vi "ADC SNR_input_sweep.vi"(8 "error in (no error)":errorcluster, 9 "Sequence parameters":string[][](array[string])=[["Min limit", "Max limit", "Register sheet file", "Register Sheet"], ["", "", "CC2600.xls", "TX_BLE;Trim"], ["Reg write (addr;value)", "Operating frequency [Hz]", "", ""], ["NA", "2.44G", "", ""]], 10 "Run type":i32, 11 "Method parameters":T3={"Dev"={"Do not disturb DUT"=FALSE, "XOSC"=32000000.0, "Board type"="", "EM"="", "Configure tempboard"=TRUE, "Device specific info"=[], "Generic Object"=refnum}, "Method"={"Run type"=1, "Test name"="Current LPM2 4", "Comment"="", "Results folder"="", "AFC"=enum."Off", "Method name"="Current LPM2 4", "Method results"={"Excel brief report"=FALSE, "Spotfire report"=FALSE, "Starfish report"=FALSE}, "Operator"="", "Reference time"=timestamp(0 s since 1904-01-01), "AFC delay"=0.0, "Initialization"=enum."Enabled", "MD5 Sum"="", "HW addon board"=enum."None", "AFC Regsheet"="", "AFC Regfile"=path "", "dummy"=0.0}, "Inst"={"Instr"={"PS1"={"Name"="", "GPIB address"="", "VISA session"=""}, "PS2"={"Name"="", "GPIB address"="", "VISA session"=""}, "TC1"={"Name"="", "GPIB address"="", "VISA session"=""}, "TC2"={"Name"="", "GPIB address"="", "VISA session"=""}, "SA1"={"Name"="", "GPIB address"="", "VISA session"=""}, "SA2"={"Name"="", "GPIB address"="", "VISA session"=""}, "SG1"={"Name"="", "GPIB address"="", "VISA session"=""}, "SG2"={"Name"="", "GPIB address"="", "VISA session"=""}, "SG3"={"Name"="", "GPIB address"="", "VISA session"=""}, "MI1"={"Name"="", "GPIB address"="", "VISA session"=""}, "MI2"={"Name"="", "GPIB address"="", "VISA session"=""}, "SW SA"={"Name"="", "Controller addr"=""}, "SW SG"={"Name"="", "Controller addr"=""}, "MI3"={"Name"="", "GPIB address"="", "VISA session"=""}}, "Switchbox"={"RF Path"=0, "Cal compensation"=enum."TX", "Switchbox gain mode"="", "State"=enum."TX"}, "Instr to control (i.e. SA1)"="Default", "Intrument info string"=""}, "Sequence parameters"=[["Weight", "Min Limit", "Max Limit", "Register Sheet", "", "", "", "", "", "", "", "", ""], ["Vital", "", "1", "LPM2", "", "", "", "", "", "", "", "", ""], ["Resolution", "Reg write (addr;value)", "Chip mode", "Range", "", "", "", "", "", "", "", "", ""], ["u", "NA", "", "auto", "", "", "", "", "", "", "", "", ""]], "Cond"={"Temp logged"=25.0, "VDD1_PS1_6V"=-999.0, "VDD2_PS1_25V"=-999.0, "VDD4_PS2_25V"=-999.0, "VDD3_PS2_6V"=-999.0}, "Meas config"={"X-axis inner loop index"=32000000, "Y-axis outer loop index"=32000000, "X-axis"=[], "Y-axis"=[], "X-axis array req size"=32000000, "Y-axis array req size"=32000000, "Param description"=[], "Use meas clust for reporting"=FALSE, "Parameter index (page)"=0, "X-axis name"="", "Y-axis name"=""}} {"Cond"."VDD3_PS2_6V" format="%.3f"; "Cond"."VDD4_PS2_25V" format="%.3f"; "Cond"."VDD2_PS1_25V" format="%.3f"; "Cond"."VDD1_PS1_6V" format="%.3f"; "Method"."dummy" format="%.1p"; "Method"."AFC delay" format="%.1p"; "Dev"."XOSC" format="%.3p"}) -> (0 "error out":errorcluster, 1 "End method error":T2, 2 "Short Results":string[](array[string])=["0.00", "0.00", "0.00", "0.00"], 3 "Result summary":string[][](array[string])=[["Critical", "Output Power@2405 MHz", "-3", "4", "dBm"], ["Critical", "Output Power@2410 MHz", "-3", "4", "dBm"]])   [LabVIEW 2019]
doc: "[AutoDocStart]Performs crystal accuracy measurements. Measures the offset from ideal frequency. Primarily used for tuning XOSC capacitors and verifying XOSC trims.\n\nSweeping parameters: operating frequency, OSC override value and VDDR level\n\nResults: Offset frequency in ppm[AutoDocEnd]"
uses:
  User Lib/Utilities/Cluster definitions/Method input.ctl
  User Lib/Utilities/Cluster definitions/Device specific info.ctl
  User Lib/Utilities/Controls/Automatic Frequency Compensation types.ctl
  User Lib/Utilities/Controls/Method Reports.ctl
  User Lib/Utilities/Cluster definitions/Method Initialization.ctl
  User Lib/Utilities/Controls/HW addon boards.ctl
  User Lib/Utilities/Cluster definitions/Instr clust.ctl
  User Lib/Utilities/Switchbox control/SwitchBox_State._ENUMctl.ctl
  User Lib/Utilities/Cluster definitions/End method error cluster.ctl
  User Lib/Utilities/Cluster definitions/DUT vdd control.ctl
  User Lib/Utilities/Cluster definitions/DUT VDD4.ctl
  User Lib/Utilities/Cluster definitions/DUT VDD3.ctl
  User Lib/Utilities/Cluster definitions/DUT VDD2.ctl
  User Lib/Utilities/Cluster definitions/DUT VDD1.ctl
  35ec0895-51f9-4de3-b2a6-381c8b522c68.vi
  a1a5dd50-ef75-4989-863a-e44a6a63b90e.vi
  3a26386c-adf8-4bfd-9313-23d3b8777f38.vi
panel:
  in  "Tab Control":T1(tab)
  # "°C"
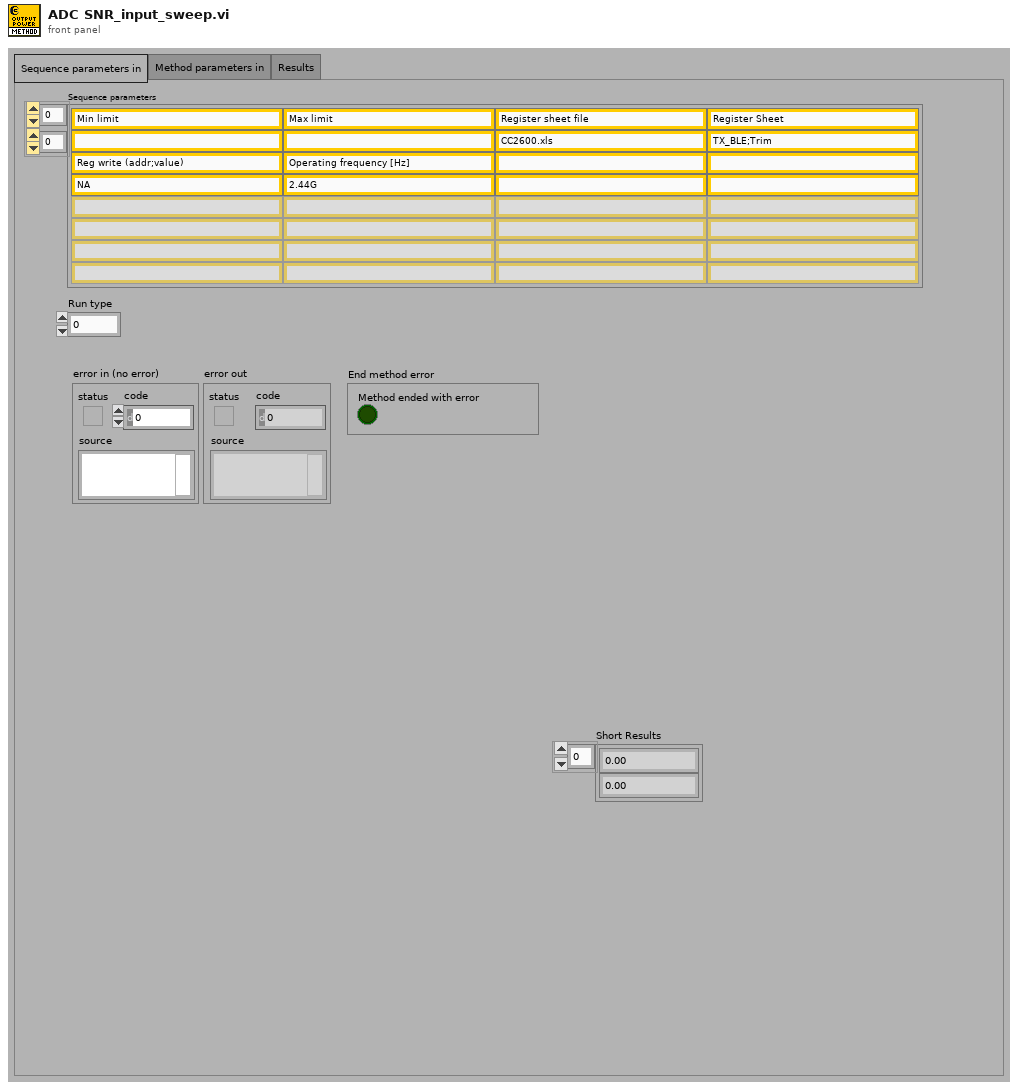
[diagram p1: front panel]
types:
  T1 = enum32{"Sequence parameters in", "Method parameters in", "Results"}
  T2 = typedef "End method error cluster.ctl" = cluster{"Method ended with error":bool}
  T3 = typedef "Method input.ctl" = cluster{"Dev":cluster{"Do not disturb DUT":bool, "XOSC":dbl, "Board type":string, "EM":string, "Configure tempboard":bool, "Device specific info":T4[], "Generic Object":refnum<class>}, "Method":cluster{"Run type":i32, "Test name":string, "Comment":string, "Results folder":string, "AFC":T5, "Method name":string, "Method results":T6, "Operator":string, "Reference time":timestamp, "AFC delay":dbl, "Initialization":T7, "MD5 Sum":string, "HW addon board":T8, "AFC Regsheet":string, "AFC Regfile":path, "dummy":dbl}, "Inst":T9, "Sequence parameters":string[][], "Cond":cluster{"Temp logged":dbl, "VDD1_PS1_6V":dbl, "VDD2_PS1_25V":dbl, "VDD4_PS2_25V":dbl, "VDD3_PS2_6V":dbl}, "Meas config":cluster{"X-axis inner loop index":i32, "Y-axis outer loop index":i32, "X-axis":string[], "Y-axis":string[], "X-axis array req size":i32, "Y-axis array req size":i32, "Param description":string[][], "Use meas clust for reporting":bool, "Parameter index (page)":i32, "X-axis name":string, "Y-axis name":string}}
  T4 = typedef "Device specific info.ctl" = cluster{"EM number":u8, "IP address":string, "Enabled":bool, "Slot no":u8, "RF path":u8, "EM name":string, "Wafer info":string, "AFC frequency ppm":dbl, "Register writes":string[][], "Meas data":string[][][], "Device comment":string}
  T5 = typedef "Automatic Frequency Compensation types.ctl" = enum16{"Off", "Compensate Instrument frequency", "Compensate DUT frequency", "Predictive - Compensate Instrument frequency", "Predictive - Compensate DUT frequency", "Do not skip re-init - Compensate Instrument frequency", "Do not skip re-init - Compensate DUT frequency"}
  T6 = typedef "Method Reports.ctl" = cluster{"Excel brief report":bool, "Spotfire report":bool, "Starfish report":bool}
  T7 = typedef "Method Initialization.ctl" = enum16{"Enabled", "Skip Instr and Device Init", "Enabled with Separate Flash", "Set PS, Device Init and Skip Instr Init", "Skip Device Init"}
  T8 = typedef "HW addon boards.ctl" = enum16{"None", "Current meas 5EM", "Stresstest 10EM"}
  T9 = typedef "Instr clust.ctl" = cluster{"Instr":cluster{"PS1":cluster{"Name":string, "GPIB address":string, "VISA session":refnum<visa-resource-name>}, "PS2":cluster{"Name":string, "GPIB address":string, "VISA session":refnum<visa-resource-name>}, "TC1":cluster{"Name":string, "GPIB address":string, "VISA session":refnum<visa-resource-name>}, "TC2":cluster{"Name":string, "GPIB address":string, "VISA session":refnum<visa-resource-name>}, "SA1":cluster{"Name":string, "GPIB address":string, "VISA session":refnum<visa-resource-name>}, "SA2":cluster{"Name":string, "GPIB address":string, "VISA session":refnum<visa-resource-name>}, "SG1":cluster{"Name":string, "GPIB address":string, "VISA session":refnum<visa-resource-name>}, "SG2":cluster{"Name":string, "GPIB address":string, "VISA session":refnum<visa-resource-name>}, "SG3":cluster{"Name":string, "GPIB address":string, "VISA session":refnum<visa-resource-name>}, "MI1":cluster{"Name":string, "GPIB address":string, "VISA session":refnum<visa-resource-name>}, "MI2":cluster{"Name":string, "GPIB address":string, "VISA session":refnum<visa-resource-name>}, "SW SA":cluster{"Name":string, "Controller addr":string}, "SW SG":cluster{"Name":string, "Controller addr":string}, "MI3":cluster{"Name":string, "GPIB address":string, "VISA session":refnum<visa-resource-name>}}, "Switchbox":cluster{"RF Path":i32, "Cal compensation":enum16{"TX", "RX", "Interferer", "No compensation", "Interferer2"}, "Switchbox gain mode":string, "State":T10}, "Instr to control (i.e. SA1)":string, "Intrument info string":string}
  T10 = typedef "SwitchBox_State._ENUMctl.ctl" = enum16{"TX", "RX", "SP:TX", "SP:RX", "SW:TX", "SW:RX"}
  T11 = typedef "DUT vdd control.ctl" = cluster{"VDD4 config":T12, "VDD3 config":T13, "VDD2 config":T14, "VDD1 config":T15}
  T12 = typedef "DUT VDD4.ctl" = u16
  T13 = typedef "DUT VDD3.ctl" = u16
  T14 = typedef "DUT VDD2.ctl" = u16
  T15 = typedef "DUT VDD1.ctl" = u16
  T16 = cluster{"Fundamental Frequency":dbl, "Sampling Frequncy":dbl, "No of Harmonics":u8, "Window":enum16{"None ", "Hanning", "Hamming", "Blackman-Harris", "Exact Blackman", "Blackman", "Flat Top", "4 Term B-Harris ", "7 Term B-Harris"}, "Blackman (fundamental power) bins)":dbl}
  T17 = enum32{"NI Card Settings", "Memory Read Setting", "DC Capture", "ADC Ramp", "ADC Sine", "SNR", "Cap Calibration"}
  T18 = enum32{"Read from Memory", "Read .dat file", "NI Card Capture", "None"}
  T19 = cluster{"Path to Save plot":path, "Path to Raw Data plot":path}
  T20 = cluster{"Save INL/DNL Plot(Ramp)":bool, "Save SNR Plot":bool, "Save INL/DNL Plot(Sine)":bool, "Save INL/DNL Raw Data(Ramp)":bool, "Save SNR Raw Data":bool, "Save INL/DNL Raw Data(Sine)":bool, "Save DC Raw data":bool, "Save  Raw Data(Sine)":bool}
  T21 = cluster{"SNR":dbl, "SNRD":dbl, "THD":dbl, "ENOB (SNRD)":dbl, "SFDR":dbl, "ENOB (SNR)":dbl, "Noise Power":dbl, "Signal power":dbl}
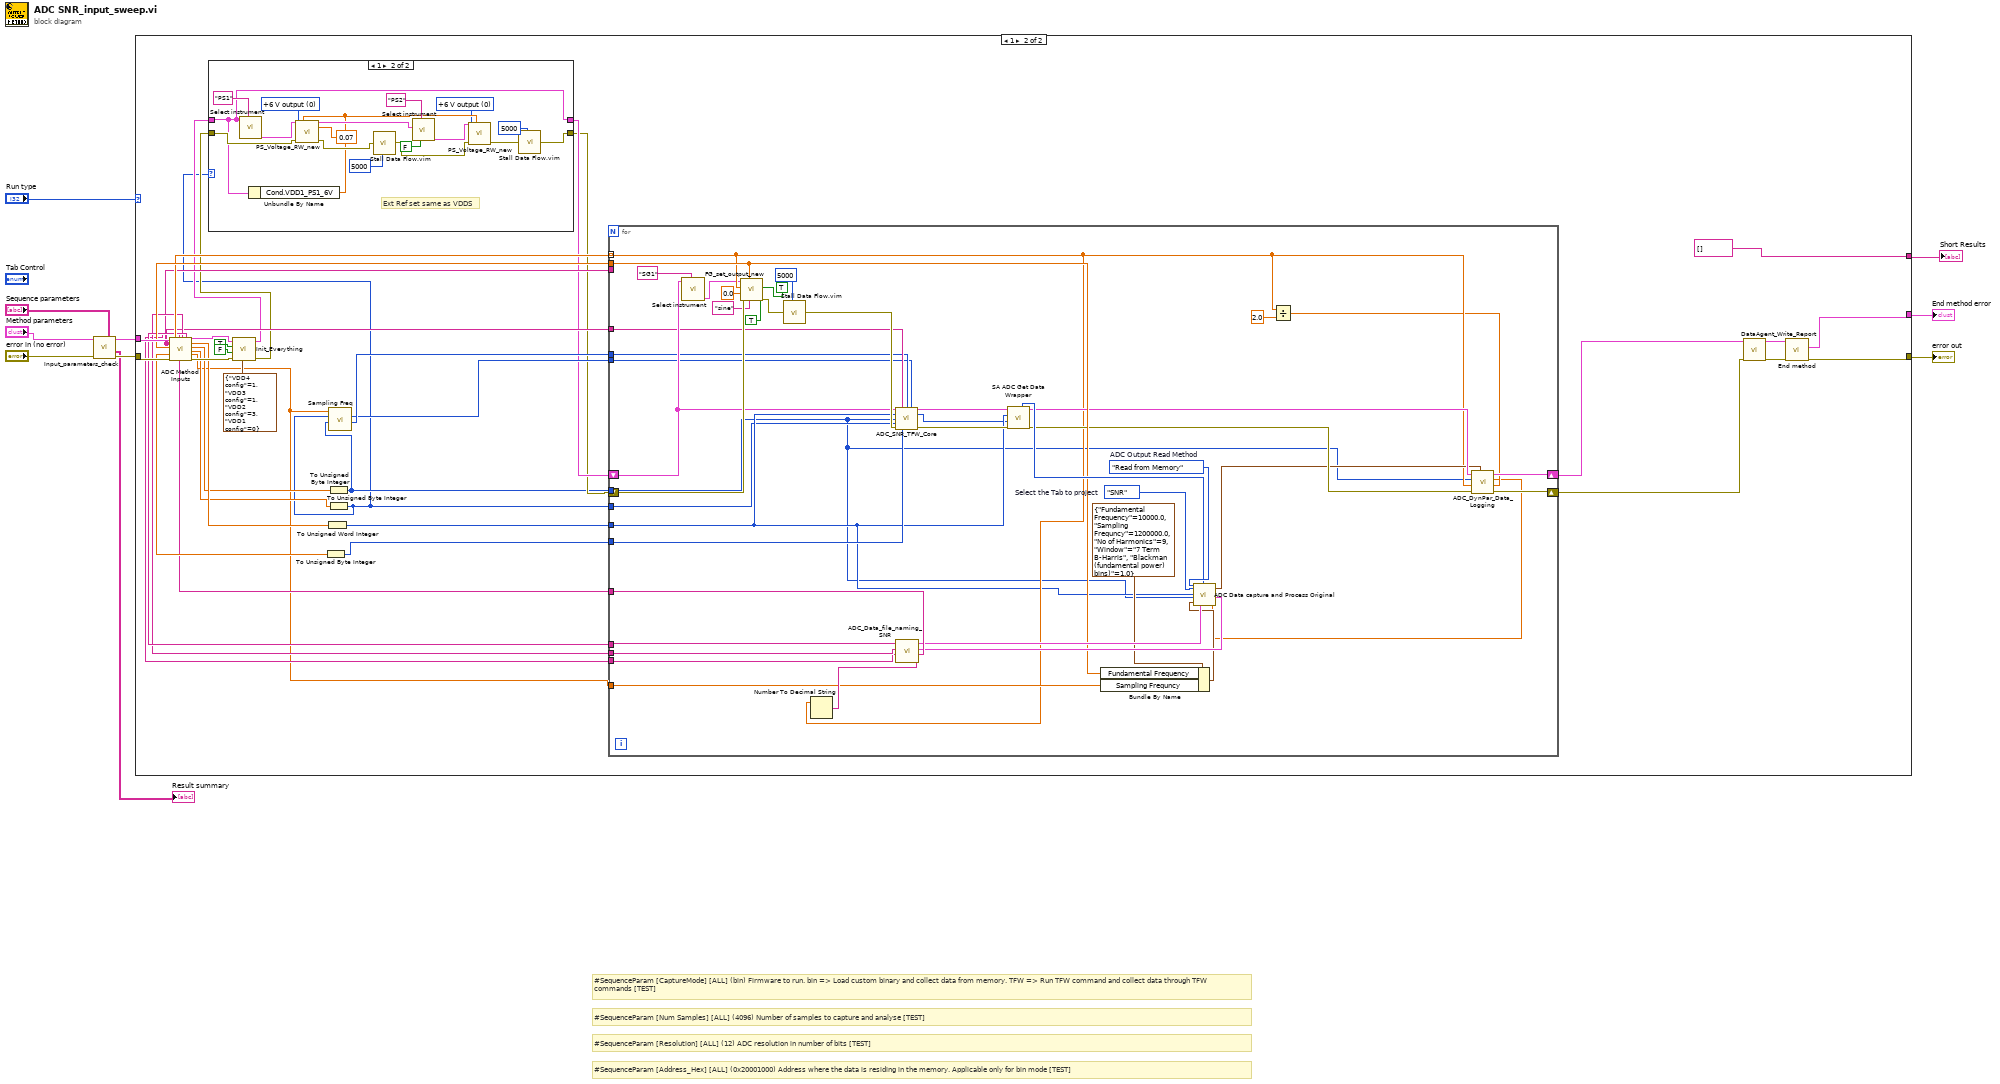
[diagram p0: block diagram]
diagram:
  # "#SequenceParam [Num Samples] [ALL] (4096) Number of samples to capture and analyse [TEST]"
  # "#SequenceParam [CaptureMode] [ALL] (bin) Firmware to run. bin => Load custom binary and collect data from memory. TFW => Run TFW command and collect data through TFW commands [TEST]"
  # "#SequenceParam [Address_Hex] [ALL] (0x20001000) Address where the data is residing in the memory. Applicable only for bin mode [TEST]"
  # "#SequenceParam [Resolution] [ALL] (12) ADC resolution in number of bits [TEST]"
  n1 = call "Input_parameters_check.vi"("Sequence parameters"="Sequence parameters", "error in"="error in (no error)", "Method cluster in"="Method parameters") -> ("error out"=w9:errorcluster, "Result summary"=→"Result summary":string[][], "Method cluster out"=w5:T3)  [unwired: 6 in]
  n2 = case shown="1" "Run type" {
    tunnel: w9 -> [w11 w36]
    tunnel: [w11 w47] -> w10
    tunnel: w5 -> [_ w37]
    tunnel: [_ w46] -> w4
    tunnel: [_ string[] []] -> w1
    frame 0, Default {
      # "Run type 0 is only for formatting the result summary"
    }
    frame 1 {
      n3 = call "ADC Method Inputs.vi"("Method cluster in"=w37, "error in (no error)"=w36) -> ("Capture Mode"=w18:string, "Signal Freq"=w25:dbl, "ADC Chnl No."=w30:dbl, "Input Voltage"=w24:dbl[], "Sampling Freq String"=w21:string, "Chnl No. string"=w20:string, "Resolution String"=w22:string, "Voltage Ref String"=w23:string, "Method cluster out"=w34:T3, "Num Samples"=w33:dbl, "Resolution"=w32:dbl, "Voltage Ref"=w31:dbl, "Sampling Freq"=w19:dbl, "error out"=w35:errorcluster)  [unwired: 3 in, 1 out]
      n4 = call "Init_Everything.vi"("VDD config"=T11 {"VDD4 config"=1, "VDD3 config"=1, "VDD2 config"=3, "VDD1 config"=0}, "error in"=w35, "Support current measurement?"=FALSE, "Override VDD Config"=TRUE, "Method cluster In"=w34) -> ("error out"=w16:errorcluster, "Method cluster out"=w17:T3)  [unwired: 3 in, 2 out]
      n5 = To Unsigned Byte Integer(number=w30) -> (unsigned 8bit integer=w28:u8)
      n6 = To Unsigned Word Integer(number=w33) -> (unsigned 16bit integer=w29:u16)
      n7 = To Unsigned Byte Integer(number=w32) -> (unsigned 8bit integer=w13:u8)
      n8 = To Unsigned Byte Integer(number=w31) -> (unsigned 8bit integer=w12:u8)
      n9 = case shown="1" w12 {
        tunnel: w17 -> [w49 w54]
        tunnel: [w49 w54] -> w15
        tunnel: w16 -> [w48 w62]
        tunnel: [w48 w52] -> w14
        frame 0, 2, 3, Default {
        }
        frame 1 {
          w50 = u16 0 items=["+6 V output", "+25 V output", "-25 V output", "ALL TERM"] ("Output Terminals")
          w65 = u16 0 items=["+6 V output", "+25 V output", "-25 V output", "ALL TERM"] ("Output Terminals")
          # "Ext Ref set same as VDDS"
          n10 = call "Select instrument.vi"("Instr.Instr to control (i.e. SA1)"="PS1", "Method cluster in"=w54) -> ("Instr out"=w66:T9)  [unwired: 7 in, 2 out]
          n11 = Unbundle By Name(w54) -> ("Cond.VDD1_PS1_6V"=w56:dbl)
          n12 = call "PS_Voltage_RW_new.vi"("InstrCluster in"=w66, "Set Voltage"=w56, "Current(0)"=0.07, "Output Terminals"=w65, "error in (no error)"=w62) -> ("InstrCluster out"=w60:T9, "error out"=w63:errorcluster)  [unwired: 8 in, 1 out]
          n13 = call "Stall Data Flow.vim"("value in"=w63, "milliseconds to wait"=u32 5000) -> ("value out"=w55:errorcluster)  [unwired: 1 out]
          n14 = call "Select instrument.vi"("Method cluster (T) / Instr cluster (F)"=FALSE, "Instr.Instr to control (i.e. SA1)"="PS2", "Instr in"=w60) -> ("Instr out"=w57:T9)  [unwired: 6 in, 2 out]
          n15 = call "PS_Voltage_RW_new.vi"("InstrCluster in"=w57, "Set Voltage"=w56, "Output Terminals"=w50, "error in (no error)"=w55) -> ("error out"=w53:errorcluster)  [unwired: 9 in, 2 out]
          n16 = call "Stall Data Flow.vim"("value in"=w53, "milliseconds to wait"=u32 5000) -> ("value out"=w52:errorcluster)  [unwired: 1 out]
        }
      }
      n17 = call "Sampling Freq.vi"("Resolution"=w13, "Voltage Ref"=w12, "Sampling Freq"=w19) -> ("LGPT Count"=w27:u16, "SCOMP"=w26:u16)  [unwired: 7 in]
      n18 = for {
        tunnel: w29 -> [w82]
        tunnel: w13 -> [w80]
        tunnel: w12 -> [w81]
        tunnel: w28 -> [w83]
        tunnel: w18 -> [_]
        tunnel: w27 -> [w78]
        tunnel: w26 -> [w77]
        shift-right: [w95] -> w41
        shift-left: w15 -> [w84]
        shift-right: [w94] -> w40
        shift-left: w14 -> [w111]
        tunnel: w24 -> [w90] mode=indexing
        tunnel: w25 -> [w97]
        tunnel: w23 -> [w108]
        tunnel: w22 -> [w107]
        tunnel: w21 -> [w106]
        tunnel: w20 -> [w109]
        tunnel: w19 -> [w96]
        tunnel: w18 -> [w79]
        w101 = T17."SNR"  # Select the Tab to project
        w102 = T18."Read from Memory"  # ADC Output Read Method
        n19 = call "Select instrument.vi"("Instr.Instr to control (i.e. SA1)"="SG1", "Method cluster in"=w84) -> ("Instr out"=w75:T9)  [unwired: 7 in, 2 out]
        n20 = call "FG_set_output_new.vi"("High impedance (T)"=TRUE, "Enable Output?"=TRUE, "Function (DC, Sine, Square, Triangle, Ramp up, Ramp down, Pulse)"="sine", "Frequency [Hz]"=w97, "error in"=w111, "Low voltage"=0.0, "High voltage (or DC)"=w90, "InstrCluster in"=w75) -> ("error out"=w73:errorcluster)  [unwired: 2 in, 1 out]
        n21 = call "Stall Data Flow.vim"("value in"=w73, "milliseconds to wait"=u32 5000) -> ("value out"=w85:errorcluster)  [unwired: 1 out]
        n22 = Number To Decimal String(number=w90) -> (decimal integer string=w103:string)  [unwired: 1 in]
        n23 = call "ADC_SNR_TFW_Core.vi"("Method cluster in"=w84, "Capture Mode"=w79, "LGPT Count"=w78, "SCOMP"=w77, "No. Samples"=w82, "Resolution"=w80, "Voltage Ref"=w81, "error in"=w85, "ADC Chnl No."=w83) -> ("Method cluster out 2"=w87:T3, "ResPar[0] Data Address"=w76:u32, "error out"=w86:errorcluster)  [unwired: 3 in, 1 out]
        n24 = call "ADC_Data_file_naming_SNR.vi"("Amplitude (Vpp)"=w103, "ADC Chn. No"=w109, "Sampling Freq String"=w106, "Resolution String"=w107, "Voltage Ref String"=w108) -> ("path to save"=w104:T19, "Save data"=w105:T20)  [unwired: 5 in]
        n25 = call "SA ADC Get Data Wrapper.vi"("error in"=w86, "Data Address"=w76, "Num Samples"=w82, "Method cluster in"=w87) -> ("error out"=w92:errorcluster, "output cluster"=w93:T3, "ADC samples"=w100:u32[])  [unwired: 2 in, 3 out]
        n26 = Bundle By Name(cluster=T16 {"Fundamental Frequency"=10000.0, "Sampling Frequncy"=1200000.0, "No of Harmonics"=9, "Window"=enum."7 Term B-Harris", "Blackman (fundamental power) bins)"=1.0} ("Inputs for Dyanmic para"), "Fundamental Frequency"=w97, "Sampling Frequncy"=w96) -> (w98:T16)
        n27 = call "ADC Data capture and Process Original.vi"("ADC Output Read Method"=w102, "Select the Tab to project"=w101, "No.of samples(SNR)"=w82, "Resolution"=w80, "Inputs for Dyanmic para"=w98, "Save data"=w105, "Waveform"=w100, "path to save"=w104) -> ("detected Throughput"=w88:dbl, "Dynamic Parameters"=w91:T21)  [unwired: 13 in, 5 out]
        n28 = Divide(x=w90, y=2.0) -> (x/y=w89:dbl)
        n29 = call "ADC_DynPar_Data_Logging.vi"("Offset (V)"=w89, "detected Throughput"=w88, "Dynamic Parameters"=w91, "error in (no error)"=w92, "Amplitude (Vpp)"=w90, "Ref Voltage"=w80, "Method cluster in"=w93) -> ("error out"=w94:errorcluster, "Method cluster out"=w95:T3)  [unwired: 3 in]
      }
      n30 = call "DataAgent_Write_Report.vi"("error in (no error)"=w40, "Method cluster in"=w41) -> ("error out"=w44:errorcluster, "Method cluster out"=w43:T3)  [unwired: 8 in]
      n31 = call "End method.vi"("error in"=w44, "Method cluster in"=w43) -> ("error out"=w47:errorcluster, "End method error"=w46:T2)  [unwired: 7 in, 1 out]
    }
  }
  "error out" <- w10
  "End method error" <- w4
  "Short Results" <- w1
